vi "checkoffWaypoints.vi"(10 "Mission QueueRef":T1, 11 "NotifierReff":T2) -> (2 "Waypoints Queue Out":refnum<queue>, 3 "BoatLocation Notifier Out":refnum<notifier>)   [LabVIEW 2013]
doc: "Removes waypoint from Queue if it's been checked off AND if there's still at least one element in the queue\n\n-Kaitlin (3/12/14)"
uses:
  Data/TypeDefs/Notifiers.ctl
  Data/TypeDefs/UTM Location.ctl
  Data/TypeDefs/Sail Set Suggestions.ctl
  Data/TypeDefs/Rudder Set Suggestions.ctl
  Data/TypeDefs/OverrideInformation.ctl
  Data/TypeDefs/OverrideMode.ctl
  Data/TypeDefs/MotorSetup.ctl
  Data/TypeDefs/DynamixelSetupInfo.ctl
  Data/TypeDefs/AirmarStatus.ctl
  Data/TypeDefs/HardwareOnline.ctl
  Data/TypeDefs/DynamixelCycleTracker.ctl
  Data/TypeDefs/Queues.ctl
  Classes/Waypoint/Waypoint.lvclass
  Classes/Missions/GenericMission/GenericMission.lvclass
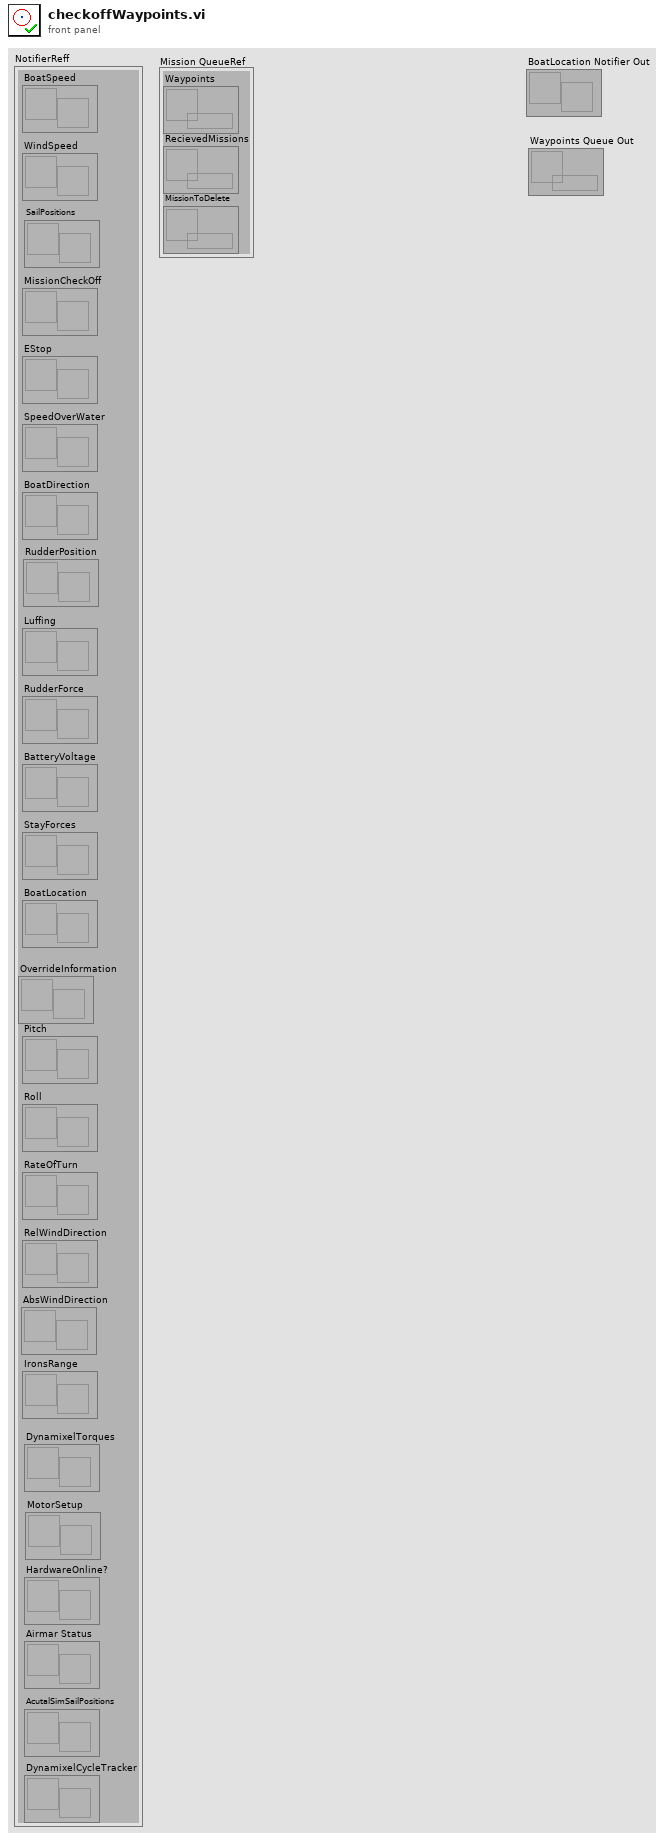
[diagram p1: front panel]
types:
  T1 = typedef "Queues.ctl" = cluster{"Waypoints":refnum<queue>, "RecievedMissions":refnum<queue>, "MissionToDelete":refnum<queue>}
  T2 = typedef "Notifiers.ctl" = cluster{"BoatSpeed":refnum<notifier>, "WindSpeed":refnum<notifier>, "MissionCheckOff":refnum<notifier>, "EStop":refnum<notifier>, "SpeedOverWater":refnum<notifier>, "BoatDirection":refnum<notifier>, "Luffing":refnum<notifier>, "RudderForce":refnum<notifier>, "BatteryVoltage":refnum<notifier>, "StayForces":refnum<notifier>, "BoatLocation":refnum<notifier>, "Pitch":refnum<notifier>, "Roll":refnum<notifier>, "RateOfTurn":refnum<notifier>, "RelWindDirection":refnum<notifier>, "SailPositions":refnum<notifier>, "RudderPosition":refnum<notifier>, "IronsRange":refnum<notifier>, "AbsWindDirection":refnum<notifier>, "OverrideInformation":refnum<notifier>, "DynamixelTorques":refnum<notifier>, "MotorSetup":refnum<notifier>, "Airmar Status":refnum<notifier>, "HardwareOnline?":refnum<notifier>, "AcutalSimSailPositions":refnum<notifier>, "DynamixelCycleTracker":refnum<notifier>}
  T3 = typedef "UTM Location.ctl" = cluster{"UTM Zone":dbl, "Hemisphere":enum16{"North", "South"}, "East":dbl, "North":dbl}
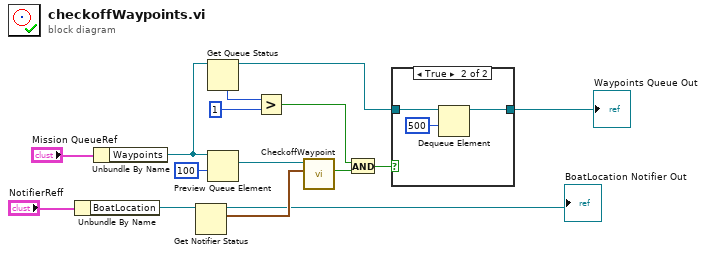
[diagram p0: block diagram]
diagram:
  n1 = Unbundle By Name("NotifierReff") -> ("BoatLocation"=w14:refnum<notifier>)
  n2 = Unbundle By Name("Mission QueueRef") -> ("Waypoints"=w7:refnum<queue>)
  n3 = Get Notifier Status(notifier=w14) -> (notifier out=→"BoatLocation Notifier Out":refnum<notifier>, current notification=w11:T3)  [unwired: 1 in, 3 out]
  n4 = Get Queue Status(queue=w7) -> (queue out=w6:refnum<queue>, # elements in queue=w5:i32)  [unwired: 2 in, 6 out]
  n5 = Preview Queue Element(queue=w7, timeout in ms (-1)=100) -> (element=w10:refnum<class "Waypoint.lvclass">)  [unwired: 1 in, 3 out]
  n6 = Greater?(x=w5, y=1) -> (0:w2:bool)
  n7 = call "CheckoffWaypoint.vi"("CurrentLocation"=w11, "Waypoint In"=w10) -> ("Done?"=w3:bool)  [unwired: 7 in, 2 out]
  n8 = And(x=w2, y=w3) -> (x .and. y?=w1:bool)
  n9 = case shown="True" w1 {
    tunnel: w6 -> [w16 w19]
    tunnel: [w16 w18] -> w9
    frame False {
    }
    frame True {
      n10 = Dequeue Element(queue=w19, timeout in ms (-1)=500) -> (queue out=w18:refnum<queue>)  [unwired: 1 in, 3 out]
    }
  }
  "Waypoints Queue Out" <- w9
